vi "Module Name--constant.vi"() -> (3 "Module Name":string)   [LabVIEW 2018, in "PLC_Launcher.lvlib"]
doc: "Return the name of the module that owns this VI. \n_____\nBased on DQMH Project Template 6.0.0.91."
uses:
  PLC_Launcher.lvlib
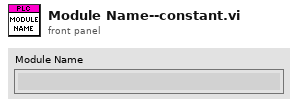
[diagram p1: front panel]
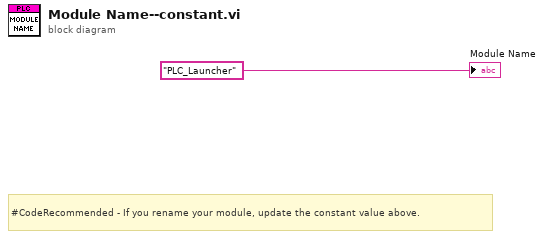
[diagram p0: block diagram]
diagram:
  # "#CodeRecommended - If you rename your module, update the constant value above."
  "Module Name" <- "PLC_Launcher"
